vi "nanocal -- nuclear schottky fit -- 2x2 -- V9.vi"() -> ()   [LabVIEW 2021] (continued)
  in  "filenames":u16(ring)=29 caption="files" items=["IDS0183_210310_RAW_cal_CeCoIn5_2nd_071_12T_0.120K_90deg_Tdep_raw_.dat", "IDS0311_210901_RAW_cal_CeCoIn5_4th_040(126)_C(f)_12T_0.120K_45deg_Tdep_raw_.dat", "IDS0359_210907_RAW_cal_CeCoIn5_4th_089_C(f)_12.0T_0.12K_60deg_Tdep_raw_.dat", "IDS0412_220525_RAW_cal_CeCoIn5_5th_017_0T_0deg__fSweep_0.12K_raw_.dat", "IDS0431_220527_RAW_cal_CeCoIn5_5th_036_10T_0deg__fSweep_0.12K_raw_.dat", "IDS0442_220528_RAW_cal_CeCoIn5_5th_047_6T_0deg__fSweep_0.12K_raw_.dat", "IDS0464_220530_RAW_cal_CeCoIn5_5th_069_4T_0deg__fSweep_0.12K_raw_.dat", "IDS0486_220602_RAW_cal_CeCoIn5_5th_091_10T_45deg__fSweep_0.12K_raw_.dat", "IDS0336_210904_RAW_cal_CeCoIn5_4th_065_C(f)_5.0T_0.122K_90deg_Tdep_raw_.dat", "IDS0346_210904_RAW_cal_CeCoIn5_4th_075_C(f)_8.0T_0.122K_90deg_Tdep_raw_.dat", "IDS0378_210909_RAW_cal_CeCoIn5_4th_108_C(f)_8.0T_0.122K_0deg_Tdep_raw_.dat", "IDS0158_210310_RAW_cal_CeCoIn5_2nd_047_12T_fsweep_final_0.14K_0deg_Tdep_raw_.dat", "IDS0300_210427_RAW_cal_CeCoIn5_4th_029(113)_C(f)_12T_0.14K_30deg_NEW_Tdep_raw_.dat", "IDS0184_210310_RAW_cal_CeCoIn5_2nd_072_12T_0.148K_90deg_Tdep_raw_.dat", "IDS0210_210310_RAW_cal_CeCoIn5_2nd_098_fsweep_6T_0.148K_Bdep_raw_.dat", "IDS0379_210909_RAW_cal_CeCoIn5_4th_109_C(f)_8.0T_0.148K_0deg_Tdep_raw_.dat", "IDS0360_210907_RAW_cal_CeCoIn5_4th_090_C(f)_12.0T_0.15K_60deg_Tdep_raw_.dat", "IDS0411_220525_RAW_cal_CeCoIn5_5th_016_0T_0deg__fSweep_0.15K_raw_.dat", "IDS0427_220526_RAW_cal_CeCoIn5_5th_032_10T_0deg__fSweep_0.15K_raw_.dat", "IDS0443_220528_RAW_cal_CeCoIn5_5th_048_6T_0deg__fSweep_0.15K_raw_.dat", "IDS0463_220530_RAW_cal_CeCoIn5_5th_068_4T_0deg__fSweep_0.15K_raw_.dat", "IDS0487_220602_RAW_cal_CeCoIn5_5th_092_10T_45deg__fSweep_0.15K_raw_.dat", "IDS0310_210901_RAW_cal_CeCoIn5_4th_039(125)_C(f)_12T_0.157K_45deg_Tdep_raw_.dat", "IDS0337_210904_RAW_cal_CeCoIn5_4th_066_C(f)_5.0T_0.157K_90deg_Tdep_raw_.dat", "IDS0347_210906_RAW_cal_CeCoIn5_4th_076_C(f)_8.0T_0.157K_90deg_Tdep_raw_.dat", "IDS0305_210831_RAW_cal_CeCoIn5_4th_034(110)_C(f)_12T_0.16K_30deg_NEW_Tdep_raw_.dat", "IDS0361_210908_RAW_cal_CeCoIn5_4th_091_C(f)_12.0T_0.168K_60deg_Tdep_raw_.dat", "IDS0380_210909_RAW_cal_CeCoIn5_4th_110_C(f)_8.0T_0.168K_0deg_Tdep_raw_.dat", "IDS0159_210310_RAW_cal_CeCoIn5_2nd_048_12T_fsweep_0.17K_0deg_Tdep_raw_.dat", "IDS0304_210831_RAW_cal_CeCoIn5_4th_033(112)_C(f)_12T_0.17K_30deg_NEW_Tdep_raw_.dat", "IDS0312_210901_RAW_cal_CeCoIn5_4th_041(127)_C(f)_12T_0.170K_45deg_Tdep_raw_.dat", "IDS0338_210904_RAW_cal_CeCoIn5_4th_067_C(f)_5.0T_0.170K_90deg_Tdep_raw_.dat", "IDS0410_220525_RAW_cal_CeCoIn5_5th_015_0T_0deg__fSweep_0.17K_raw_.dat", "IDS0432_220527_RAW_cal_CeCoIn5_5th_037_10T_0deg__fSweep_0.17K_raw_.dat", "IDS0444_220528_RAW_cal_CeCoIn5_5th_049_6T_0deg__fSweep_0.17K_raw_.dat", "IDS0462_220530_RAW_cal_CeCoIn5_5th_067_4T_0deg__fSweep_0.17K_raw_.dat", "IDS0485_220601_RAW_cal_CeCoIn5_5th_090_10T_45deg__fSweep_0.17K_raw_.dat", "IDS0348_210906_RAW_cal_CeCoIn5_4th_077_C(f)_8.0T_0.178K_90deg_Tdep_raw_.dat", "IDS0181_210310_RAW_cal_CeCoIn5_2nd_070_12T_0.179K_90deg_fsweep_Tdep_raw_.dat", "IDS0424_220526_RAW_cal_CeCoIn5_5th_029_10T_0deg__fSweep_0.19K_raw_.dat", "IDS0185_210310_RAW_cal_CeCoIn5_2nd_073_12T_0.197K_90deg_Tdep_raw_.dat", "IDS0208_210310_RAW_cal_CeCoIn5_2nd_096_Hsweep_0.197K_Bdep_raw_.dat", "IDS0209_210310_RAW_cal_CeCoIn5_2nd_097_Hsweep_0.197K_Bdep_raw_.dat", "IDS0211_210310_RAW_cal_CeCoIn5_2nd_099_fsweep_9T_0.197K_Bdep_raw_.dat", "IDS0212_210310_RAW_cal_CeCoIn5_2nd_100_fsweep_11T_0.197K_Bdep_raw_.dat", "IDS0213_210310_RAW_cal_CeCoIn5_2nd_101_fsweep_10T_0.197K_Bdep_raw_.dat", "IDS0214_210310_RAW_cal_CeCoIn5_2nd_102_fsweep_8T_0.197K_Bdep_raw_.dat", "IDS0215_210310_RAW_cal_CeCoIn5_2nd_103_fsweep_7T_0.197K_Bdep_raw_.dat", "IDS0216_210310_RAW_cal_CeCoIn5_2nd_104_fsweep_5T_0.197K_Bdep_raw_.dat", "IDS0217_210310_RAW_cal_CeCoIn5_2nd_105_fsweep_0T_0.197K_Bdep_raw_.dat", "IDS0330_210901_RAW_cal_CeCoIn5_4th_059_C(f)_1T_0.197K_90deg_Bdep_raw_.dat", "IDS0331_210901_RAW_cal_CeCoIn5_4th_060_C(f)_2T_0.197K_90deg_Bdep_raw_.dat", "IDS0335_210904_RAW_cal_CeCoIn5_4th_064_C(f)_5.0T_0.197K_90deg_Tdep_raw_.dat", "IDS0362_210908_RAW_cal_CeCoIn5_4th_092_C(f)_12.0T_0.197K_60deg_Tdep_raw_.dat", "IDS0377_210909_RAW_cal_CeCoIn5_4th_107_C(f)_8.0T_0.197K_0deg_Tdep_raw_.dat", "IDS0160_210310_RAW_cal_CeCoIn5_2nd_049_12T_fsweep_0.20K_0deg_Tdep_raw_.dat", "IDS0303_210831_RAW_cal_CeCoIn5_4th_032(114)_C(f)_12T_0.20K_30deg_NEW_Tdep_raw_.dat", "IDS0313_210901_RAW_cal_CeCoIn5_4th_042(128)_C(f)_12T_0.200K_45deg_Tdep_raw_.dat", "IDS0349_210906_RAW_cal_CeCoIn5_4th_078_C(f)_8.0T_0.20K_90deg_Tdep_raw_.dat", "IDS0407_220525_RAW_cal_CeCoIn5_5th_012_0T_0deg__fSweep_0.20K_raw_.dat", "IDS0441_220527_RAW_cal_CeCoIn5_5th_045_6T_0deg__fSweep_0.20K_raw_.dat", "IDS0458_220529_RAW_cal_CeCoIn5_5th_063_4T_0deg__fSweep_0.20K_raw_.dat", "IDS0477_220601_RAW_cal_CeCoIn5_5th_082_10T_45deg__fSweep_0.20K_raw_.dat", "IDS0161_210310_RAW_cal_CeCoIn5_2nd_050_12T_fsweep_0.22K_0deg_Tdep_raw_.dat", "IDS0186_210310_RAW_cal_CeCoIn5_2nd_074_12T_0.249K_90deg_Tdep_raw_.dat", "IDS0302_210831_RAW_cal_CeCoIn5_4th_031(115)_C(f)_12T_0.25K_30deg_NEW_Tdep_raw_.dat", "IDS0363_210908_RAW_cal_CeCoIn5_4th_093_C(f)_12.0T_0.25K_60deg_Tdep_raw_.dat", "IDS0381_210909_RAW_cal_CeCoIn5_4th_111_C(f)_8.0T_0.25K_0deg_Tdep_raw_.dat", "IDS0408_220525_RAW_cal_CeCoIn5_5th_013_0T_0deg__fSweep_0.25K_raw_.dat", "IDS0425_220526_RAW_cal_CeCoIn5_5th_030_10T_0deg__fSweep_0.25K_raw_.dat", "IDS0445_220528_RAW_cal_CeCoIn5_5th_050_6T_0deg__fSweep_0.25K_raw_.dat", "IDS0459_220529_RAW_cal_CeCoIn5_5th_064_4T_0deg__fSweep_0.25K_raw_.dat", "IDS0478_220601_RAW_cal_CeCoIn5_5th_083_10T_45deg__fSweep_0.25K_raw_.dat", "IDS0314_210901_RAW_cal_CeCoIn5_4th_043(129)_C(f)_12T_0.255K_45deg_Tdep_raw_.dat", "IDS0339_210904_RAW_cal_CeCoIn5_4th_068_C(f)_5.0T_0.255K_90deg_Tdep_raw_.dat", "IDS0350_210906_RAW_cal_CeCoIn5_4th_079_C(f)_8.0T_0.26K_90deg_Tdep_raw_.dat", "IDS0162_210310_RAW_cal_CeCoIn5_2nd_051_12T_fsweep_0.28K_0deg_Tdep_raw_.dat", "IDS0187_210310_RAW_cal_CeCoIn5_2nd_075_12T_0.300K_90deg_Tdep_raw_.dat", "IDS0301_210831_RAW_cal_CeCoIn5_4th_030(116)_C(f)_12T_0.30K_30deg_NEW_Tdep_raw_.dat", "IDS0315_210901_RAW_cal_CeCoIn5_4th_044(130)_C(f)_12T_0.300K_45deg_Tdep_raw_.dat", "IDS0382_210909_RAW_cal_CeCoIn5_4th_112_C(f)_8.0T_0.30K_0deg_Tdep_raw_.dat", "IDS0409_220525_RAW_cal_CeCoIn5_5th_014_0T_0deg__fSweep_0.30K_raw_.dat", "IDS0426_220526_RAW_cal_CeCoIn5_5th_031_10T_0deg__fSweep_0.30K_raw_.dat", "IDS0446_220528_RAW_cal_CeCoIn5_5th_051_6T_0deg__fSweep_0.30K_raw_.dat", "IDS0460_220529_RAW_cal_CeCoIn5_5th_065_4T_0deg__fSweep_0.30K_raw_.dat", "IDS0479_220601_RAW_cal_CeCoIn5_5th_084_10T_45deg__fSweep_0.30K_raw_.dat", "IDS0364_210908_RAW_cal_CeCoIn5_4th_094_C(f)_12.0T_0.307K_60deg_Tdep_raw_.dat", "IDS0340_210904_RAW_cal_CeCoIn5_4th_069_C(f)_5.0T_0.308K_90deg_Tdep_raw_.dat", "IDS0351_210906_RAW_cal_CeCoIn5_4th_080_C(f)_8.0T_0.31K_90deg_Tdep_raw_.dat", "IDS0163_210310_RAW_cal_CeCoIn5_2nd_052_12T_fsweep_0.33K_0deg_Tdep_raw_.dat", "IDS0188_210310_RAW_cal_CeCoIn5_2nd_076_12T_0.360K_90deg_Tdep_raw_.dat", "IDS0299_210427_RAW_cal_CeCoIn5_4th_028(117)_C(f)_12T_0.36K_30deg_NEW_Tdep_raw_.dat", "IDS0316_210901_RAW_cal_CeCoIn5_4th_045(131)_C(f)_12T_0.360K_45deg_Tdep_raw_.dat", "IDS0341_210904_RAW_cal_CeCoIn5_4th_070_C(f)_5.0T_0.360K_90deg_Tdep_raw_.dat", "IDS0352_210906_RAW_cal_CeCoIn5_4th_081_C(f)_8.0T_0.36K_90deg_Tdep_raw_.dat", "IDS0365_210908_RAW_cal_CeCoIn5_4th_095_C(f)_12.0T_0.36K_60deg_Tdep_raw_.dat", "IDS0383_210910_RAW_cal_CeCoIn5_4th_113_C(f)_8.0T_0.36K_0deg_Tdep_raw_.dat", "IDS0413_220525_RAW_cal_CeCoIn5_5th_018_0T_0deg__fSweep_0.36K_raw_.dat", "IDS0428_220526_RAW_cal_CeCoIn5_5th_033_10T_0deg__fSweep_0.36K_raw_.dat", "IDS0447_220528_RAW_cal_CeCoIn5_5th_052_6T_0deg__fSweep_0.36K_raw_.dat", "IDS0461_220529_RAW_cal_CeCoIn5_5th_066_4T_0deg__fSweep_0.36K_raw_.dat", "IDS0480_220601_RAW_cal_CeCoIn5_5th_085_10T_45deg__fSweep_0.36K_raw_.dat", "IDS0164_210310_RAW_cal_CeCoIn5_2nd_053_12T_fsweep_0.40K_0deg_Tdep_raw_.dat", "IDS0429_220526_RAW_cal_CeCoIn5_5th_034_10T_0deg__fSweep_0.42K_raw_.dat", "IDS0448_220528_RAW_cal_CeCoIn5_5th_053_6T_0deg__fSweep_0.42K_raw_.dat", "IDS0481_220601_RAW_cal_CeCoIn5_5th_086_10T_45deg__fSweep_0.42K_raw_.dat", "IDS0189_210310_RAW_cal_CeCoIn5_2nd_077_12T_0.430K_90deg_Tdep_raw_.dat", "IDS0298_210427_RAW_cal_CeCoIn5_4th_027(118)_C(f)_12T_0.43K_30deg_NEW_Tdep_raw_.dat", "IDS0317_210901_RAW_cal_CeCoIn5_4th_046(132)_C(f)_12T_0.43K_45deg_Tdep_raw_.dat", "IDS0366_210908_RAW_cal_CeCoIn5_4th_096_C(f)_12.0T_0.43K_60deg_Tdep_raw_.dat", "IDS0384_210910_RAW_cal_CeCoIn5_4th_114_C(f)_8.0T_0.43K_0deg_Tdep_raw_.dat", "IDS0414_220525_RAW_cal_CeCoIn5_5th_019_0T_0deg__fSweep_0.43K_raw_.dat", "IDS0465_220530_RAW_cal_CeCoIn5_5th_070_4T_0deg__fSweep_0.43K_raw_.dat", "IDS0342_210904_RAW_cal_CeCoIn5_4th_071_C(f)_5.0T_0.438K_90deg_Tdep_raw_.dat", "IDS0353_210906_RAW_cal_CeCoIn5_4th_082_C(f)_8.0T_0.438K_90deg_Tdep_raw_.dat", "IDS0165_210310_RAW_cal_CeCoIn5_2nd_054_12T_fsweep_0.48K_0deg_Tdep_raw_.dat", "IDS0190_210310_RAW_cal_CeCoIn5_2nd_078_12T_0.512K_90deg_Tdep_raw_.dat", "IDS0430_220526_RAW_cal_CeCoIn5_5th_035_10T_0deg__fSweep_0.52K_raw_.dat", "IDS0449_220528_RAW_cal_CeCoIn5_5th_054_6T_0deg__fSweep_0.52K_raw_.dat", "IDS0482_220601_RAW_cal_CeCoIn5_5th_087_10T_45deg__fSweep_0.52K_raw_.dat", "IDS0297_210427_RAW_cal_CeCoIn5_4th_026(119)_C(f)_12T_0.53K_30deg_NEW_Tdep_raw_.dat", "IDS0318_210901_RAW_cal_CeCoIn5_4th_047(133)_C(f)_12T_0.53K_45deg_Tdep_raw_.dat", "IDS0343_210904_RAW_cal_CeCoIn5_4th_072_C(f)_5.0T_0.53K_90deg_Tdep_raw_.dat", "IDS0354_210906_RAW_cal_CeCoIn5_4th_083_C(f)_8.0T_0.53K_90deg_Tdep_raw_.dat", "IDS0367_210908_RAW_cal_CeCoIn5_4th_097_C(f)_12.0T_0.53K_60deg_Tdep_raw_.dat", "IDS0385_210910_RAW_cal_CeCoIn5_4th_115_C(f)_8.0T_0.53K_0deg_Tdep_raw_.dat", "IDS0415_220525_RAW_cal_CeCoIn5_5th_020_0T_0deg__fSweep_0.53K_raw_.dat", "IDS0466_220530_RAW_cal_CeCoIn5_5th_071_4T_0deg__fSweep_0.53K_raw_.dat", "IDS0166_210310_RAW_cal_CeCoIn5_2nd_055_12T_fsweep_0.58K_0deg_Tdep_raw_.dat", "IDS0191_210310_RAW_cal_CeCoIn5_2nd_079_12T_0.610K_90deg_Tdep_raw_.dat", "IDS0296_210427_RAW_cal_CeCoIn5_4th_025(120)_C(f)_12T_0.62K_30deg_NEW_Tdep_raw_.dat", "IDS0319_210901_RAW_cal_CeCoIn5_4th_048(134)_C(f)_12T_0.62K_45deg_Tdep_raw_.dat", "IDS0344_210904_RAW_cal_CeCoIn5_4th_073_C(f)_5.0T_0.62K_90deg_Tdep_raw_.dat", "IDS0433_220527_RAW_cal_CeCoIn5_5th_038_10T_0deg__fSweep_0.62K_raw_.dat", "IDS0450_220528_RAW_cal_CeCoIn5_5th_055_6T_0deg__fSweep_0.62K_raw_.dat", "IDS0467_220530_RAW_cal_CeCoIn5_5th_072_4T_0deg__fSweep_0.62K_raw_.dat", "IDS0483_220601_RAW_cal_CeCoIn5_5th_088_10T_45deg__fSweep_0.62K_raw_.dat", "IDS0368_210908_RAW_cal_CeCoIn5_4th_098_C(f)_12.0T_0.63K_60deg_Tdep_raw_.dat", "IDS0386_210910_RAW_cal_CeCoIn5_4th_116_C(f)_8.0T_0.63K_0deg_Tdep_raw_.dat", "IDS0416_220525_RAW_cal_CeCoIn5_5th_021_0T_0deg__fSweep_0.63K_raw_.dat", "IDS0220_210310_RAW_cal_CeCoIn5_2nd_108_fsweep_0T_0.677K_Bdep_raw_.dat", "IDS0167_210310_RAW_cal_CeCoIn5_2nd_056_12T_fsweep_0.68K_0deg_Tdep_raw_.dat", "IDS0192_210310_RAW_cal_CeCoIn5_2nd_080_12T_0.810K_90deg_Tdep_raw_.dat", "IDS0434_220527_RAW_cal_CeCoIn5_5th_039_10T_0deg__fSweep_0.82K_raw_.dat", "IDS0451_220528_RAW_cal_CeCoIn5_5th_056_6T_0deg__fSweep_0.82K_raw_.dat", "IDS0468_220530_RAW_cal_CeCoIn5_5th_073_4T_0deg__fSweep_0.82K_raw_.dat", "IDS0484_220601_RAW_cal_CeCoIn5_5th_089_10T_45deg__fSweep_0.82K_raw_.dat", "IDS0295_210427_RAW_cal_CeCoIn5_4th_024(121)_C(f)_12T_0.83K_30deg_NEW_Tdep_raw_.dat", "IDS0320_210901_RAW_cal_CeCoIn5_4th_049(135)_C(f)_12T_0.83K_45deg_Tdep_raw_.dat", "IDS0355_210906_RAW_cal_CeCoIn5_4th_085_C(f)_8.0T_0.83K_90deg_Tdep_raw_.dat", "IDS0369_210908_RAW_cal_CeCoIn5_4th_099_C(f)_12.0T_0.83K_60deg_Tdep_raw_.dat", "IDS0387_210910_RAW_cal_CeCoIn5_4th_117_C(f)_8.0T_0.83K_0deg_Tdep_raw_.dat", "IDS0417_220525_RAW_cal_CeCoIn5_5th_022_0T_0deg__fSweep_0.83K_raw_.dat", "IDS0168_210310_RAW_cal_CeCoIn5_2nd_057_12T_fsweep_0.91K_0deg_Tdep_raw_.dat", "IDS0219_210310_RAW_cal_CeCoIn5_2nd_107_fsweep_0T_1.0K_Bdep_raw_.dat", "IDS0193_210310_RAW_cal_CeCoIn5_2nd_081_12T_1.1K_90deg_Tdep_raw_.dat", "IDS0418_220525_RAW_cal_CeCoIn5_5th_023_0T_0deg__fSweep_1.12K_raw_.dat", "IDS0435_220527_RAW_cal_CeCoIn5_5th_040_10T_0deg__fSweep_1.12K_raw_.dat", "IDS0452_220528_RAW_cal_CeCoIn5_5th_057_6T_0deg__fSweep_1.12K_raw_.dat", "IDS0469_220530_RAW_cal_CeCoIn5_5th_074_4T_0deg__fSweep_1.12K_raw_.dat", "IDS0488_220602_RAW_cal_CeCoIn5_5th_093_10T_45deg__fSweep_1.12K_raw_.dat", "IDS0294_210427_RAW_cal_CeCoIn5_4th_023(122)_C(f)_12T_1.13K_30deg_NEW_Tdep_raw_.dat", "IDS0321_210901_RAW_cal_CeCoIn5_4th_050(136)_C(f)_12T_1.13K_45deg_Tdep_raw_.dat", "IDS0370_210908_RAW_cal_CeCoIn5_4th_100_C(f)_12.0T_1.13K_60deg_Tdep_raw_.dat", "IDS0388_210910_RAW_cal_CeCoIn5_4th_118_C(f)_8.0T_1.13K_0deg_Tdep_raw_.dat", "IDS0169_210310_RAW_cal_CeCoIn5_2nd_058_12T_fsweep_1.23K_0deg_Tdep_raw_.dat", "IDS0391_210910_RAW_cal_CeCoIn5_4th_121_C(f)_8.0T_1.25K_0deg_Tdep_raw_.dat", "IDS0439_220527_RAW_cal_CeCoIn5_5th_044_10T_0deg__fSweep_1.28K_raw_.dat", "IDS0395_210910_RAW_cal_CeCoIn5_4th_125_C(f)_8.0T_1.31K_0deg_Tdep_raw_.dat", "IDS0392_210910_RAW_cal_CeCoIn5_4th_122_C(f)_8.0T_1.39K_0deg_Tdep_raw_.dat", "IDS0389_210910_RAW_cal_CeCoIn5_4th_119_C(f)_8.0T_1.52K_0deg_Tdep_raw_.dat", "IDS0218_210310_RAW_cal_CeCoIn5_2nd_106_fsweep_0T_1.55K_Bdep_raw_.dat", "IDS0453_220529_RAW_cal_CeCoIn5_5th_058_6T_0deg__fSweep_1.70K_raw_.dat", "IDS0194_210310_RAW_cal_CeCoIn5_2nd_082_12T_1.8K_90deg_Tdep_raw_.dat", "IDS0293_210427_RAW_cal_CeCoIn5_4th_022(123)_C(f)_12T_1.90K_30deg_NEW_Tdep_raw_.dat", "IDS0322_210901_RAW_cal_CeCoIn5_4th_051(137)_C(f)_12T_1.90K_45deg_Tdep_raw_.dat", "IDS0371_210908_RAW_cal_CeCoIn5_4th_101_C(f)_12.0T_1.90K_60deg_Tdep_raw_.dat", "IDS0390_210910_RAW_cal_CeCoIn5_4th_120_C(f)_8.0T_1.90K_0deg_Tdep_raw_.dat", "IDS0419_220525_RAW_cal_CeCoIn5_5th_024_0T_0deg__fSweep_1.90K_raw_.dat", "IDS0436_220527_RAW_cal_CeCoIn5_5th_041_10T_0deg__fSweep_1.90K_raw_.dat", "IDS0454_220529_RAW_cal_CeCoIn5_5th_059_6T_0deg__fSweep_1.90K_raw_.dat", "IDS0470_220530_RAW_cal_CeCoIn5_5th_075_4T_0deg__fSweep_1.90K_raw_.dat", "IDS0489_220602_RAW_cal_CeCoIn5_5th_094_10T_45deg__fSweep_1.90K_raw_.dat", "IDS0170_210310_RAW_cal_CeCoIn5_2nd_059_12T_fsweep_1.97K_0deg_Tdep_raw_.dat", "IDS0420_220525_RAW_cal_CeCoIn5_5th_025_0T_0deg__fSweep_2.10K_raw_.dat", "IDS0421_220525_RAW_cal_CeCoIn5_5th_026_0T_0deg__fSweep_2.30K_raw_.dat", "IDS0471_220530_RAW_cal_CeCoIn5_5th_076_4T_0deg__fSweep_2.30K_raw_.dat", "IDS0195_210310_RAW_cal_CeCoIn5_2nd_083_12T_3.0K_90deg_Tdep_raw_.dat", "IDS0472_220530_RAW_cal_CeCoIn5_5th_077_4T_0deg__fSweep_3.07K_raw_.dat", "IDS0306_210831_RAW_cal_CeCoIn5_4th_035(124)_C(f)_12T_3.10K_30deg_NEW_Tdep_raw_.dat", "IDS0323_210901_RAW_cal_CeCoIn5_4th_052(138)_C(f)_12T_3.10K_45deg_Tdep_raw_.dat", "IDS0422_220525_RAW_cal_CeCoIn5_5th_027_0T_0deg__fSweep_3.10K_raw_.dat", "IDS0437_220527_RAW_cal_CeCoIn5_5th_042_10T_0deg__fSweep_3.10K_raw_.dat", "IDS0455_220529_RAW_cal_CeCoIn5_5th_060_6T_0deg__fSweep_3.10K_raw_.dat", "IDS0490_220602_RAW_cal_CeCoIn5_5th_095_10T_45deg__fSweep_3.10K_raw_.dat", "IDS0372_210908_RAW_cal_CeCoIn5_4th_102_C(f)_12.0T_3.11K_60deg_Tdep_raw_.dat", "IDS0393_210910_RAW_cal_CeCoIn5_4th_123_C(f)_8.0T_3.11K_0deg_Tdep_raw_.dat", "IDS0171_210310_RAW_cal_CeCoIn5_2nd_060_12T_fsweep_3.19K_0deg_Tdep_raw_.dat", "IDS0196_210310_RAW_cal_CeCoIn5_2nd_084_12T_5.7K_90deg_Tdep_raw_.dat", "IDS0324_210901_RAW_cal_CeCoIn5_4th_053(139)_C(f)_12T_5.70K_45deg_Tdep_raw_.dat", "IDS0438_220527_RAW_cal_CeCoIn5_5th_043_10T_0deg__fSweep_5.70K_raw_.dat", "IDS0456_220529_RAW_cal_CeCoIn5_5th_061_6T_0deg__fSweep_5.70K_raw_.dat", "IDS0473_220531_RAW_cal_CeCoIn5_5th_078_4T_0deg__fSweep_5.70K_raw_.dat", "IDS0373_210908_RAW_cal_CeCoIn5_4th_103_C(f)_12.0T_5.75K_60deg_Tdep_raw_.dat", "IDS0394_210910_RAW_cal_CeCoIn5_4th_124_C(f)_8.0T_5.75K_0deg_Tdep_raw_.dat", "IDS0172_210310_RAW_cal_CeCoIn5_2nd_061_12T_fsweep_5.8K_0deg_Tdep_raw_.dat"]
  in  "folder":path=path "/opt/new/Dropbox/shared_AkashAndreas/paper-CeCoIn5/Original RAW data"
  in  "file pattern":string="IDS*RAW*_raw_.dat"
  in  "string IN → Math!":bool
  in  "Math→ string OUT! :s":bool
  out "string OUT":string="  \"IDS0158_210310_RAW_cal__ref_\" ->   <|    \"ζ\" -> 0.338724462580   ,  \"τ1\" -> 0.031757745266   ,  \"τS\" -> 0.247286819047   ,  \"τN\" -> 0.322740818116   ,  \"τC\" -> 0.001034291318   ,  \"κ0\" -> 0.000000000505   ,  \"mm1\" -> 0.000261080239   ,  \"mm2\" -> 0.013473055910   ,  \"mm3\" -> 0.782167842652   ,  \"T\" -> 0.140000000000   ,  \"B\" -> 12.000000000000   ,  \"θ\" -> 0.000000000000   ,  \"Reoff\" -> -114641566.265060246000   ,  \"Imoff\" -> 0.000000000000   ,  \"στ1\" -> 0.023975320210   ,  \"στS\" -> 0.076414054009   ,  \"στN\" -> 0.076454917520    |>   , \r\"IDS0158_210310_RAW_cal__sam_\" ->   <|    \"ζ\" -> 0.286336668596   ,  \"τ1\" -> 0.037477267671   ,  \"τS\" -> 0.354459287884   ,  \"τN\" -> 0.444916383639   ,  \"τC\" -> 0.001225600579   ,  \"κ0\" -> 0.000000000596   ,  \"mm1\" -> 0.000272242393   ,  \"mm2\" -> 0.016302418461   ,  \"mm3\" -> 1.050394445660   ,  \"T\" -> 0.140000000000   ,  \"B\" -> 12.000000000000   ,  \"θ\" -> 0.000000000000   ,  \"Reoff\" -> 0.000000000000   ,  \"Imoff\" -> 0.000000000000   ,  \"στ1\" -> 0.000000000000   ,  \"στS\" -> 0.000000000000   ,  \"στN\" -> 0.000000000000    |>   , \r\"IDS0159_210310_RAW_cal__ref_\" ->   <|    \"ζ\" -> 0.271267920492   ,  \"τ1\" -> 0.029985631647   ,  \"τS\" -> 0.193691005295   ,  \"τN\" -> 0.182171075098   ,  \"τC\" -> 0.001008816819   ,  \"κ0\" -> 0.000000000648   ,  \"mm1\" -> 0.000214568285   ,  \"mm2\" -> 0.015007137955   ,  \"mm3\" -> 0.493594147559   ,  \"T\" -> 0.170000000000   ,  \"B\" -> 12.000000000000   ,  \"θ\" -> 0.000000000000   ,  \"Reoff\" -> -68518072.289156615700   ,  \"Imoff\" -> 0.000000000000   ,  \"στ1\" -> 0.012908928279   ,  \"στS\" -> 0.012278249433   ,  \"στN\" -> 0.000000000000    |>   , \r\"IDS0159_210310_RAW_cal__sam_\" ->   <|    \"ζ\" -> 0.219100303741   ,  \"τ1\" -> 0.028643012604   ,  \"τS\" -> 0.279362928811   ,  \"τN\" -> 0.246156444058   ,  \"τC\" -> 0.001272401549   ,  \"κ0\" -> 0.000000000760   ,  \"mm1\" -> 0.000227975653   ,  \"mm2\" -> 0.014929571562   ,  \"mm3\" -> 0.655418694024   ,  \"T\" -> 0.170000000000   ,  \"B\" -> 12.000000000000   ,  \"θ\" -> 0.000000000000   ,  \"Reoff\" -> 0.000000000000   ,  \"Imoff\" -> 0.000000000000   ,  \"στ1\" -> 0.000000000000   ,  \"στS\" -> 0.000000000000   ,  \"στN\" -> 0.000000000000    |>   , \r\"IDS0160_210310_RAW_cal__ref_\" ->   <|    \"ζ\" -> 0.207139977904   ,  \"τ1\" -> 0.027467343957   ,  \"τS\" -> 0.117438673826   ,  \"τN\" -> 0.102057074143   ,  \"τC\" -> 0.000949663971   ,  \"κ0\" -> 0.000000000917   ,  \"mm1\" -> 0.000162053218   ,  \"mm2\" -> 0.014024936030   ,  \"mm3\" -> 0.279192111033   ,  \"T\" -> 0.200000000000   ,  \"B\" -> 12.000000000000   ,  \"θ\" -> 0.000000000000   ,  \"Reoff\" -> -40668674.698795177000   ,  \"Imoff\" -> 0.000000000000   ,  \"στ1\" -> 0.009618369087   ,  \"στS\" -> 0.007137384425   ,  \"στN\" -> 0.000000000000    |>   , \r\"IDS0160_210310_RAW_cal__sam_\" ->   <|    \"ζ\" -> 0.170488637524   ,  \"τ1\" -> 0.029234231120   ,  \"τS\" -> 0.149095458227   ,  \"τN\" -> 0.151792620275   ,  \"τC\" -> 0.001113424175   ,  \"κ0\" -> 0.000000001042   ,  \"mm1\" -> 0.000161291869   ,  \"mm2\" -> 0.013922632736   ,  \"mm3\" -> 0.368449807743   ,  \"T\" -> 0.200000000000   ,  \"B\" -> 12.000000000000   ,  \"θ\" -> 0.000000000000   ,  \"Reoff\" -> 0.000000000000   ,  \"Imoff\" -> 0.000000000000   ,  \"στ1\" -> 0.000000000000   ,  \"στS\" -> 0.000000000000   ,  \"στN\" -> 0.000000000000    |>   , \r\"IDS0161_210310_RAW_cal__ref_\" ->   <|    \"ζ\" -> 0.165651103495   ,  \"τ1\" -> 0.025219369633   ,  \"τS\" -> 0.095243887499   ,  \"τN\" -> 0.068405844588   ,  \"τC\" -> 0.001096621932   ,  \"κ0\" -> 0.000000001058   ,  \"mm1\" -> 0.000154524257   ,  \"mm2\" -> 0.013909362731   ,  \"mm3\" -> 0.203010595371   ,  \"T\" -> 0.220000000000   ,  \"B\" -> 12.000000000000   ,  \"θ\" -> 0.000000000000   ,  \"Reoff\" -> -26138554.216867461800   ,  \"Imoff\" -> 0.000000000000   ,  \"στ1\" -> 0.007587881902   ,  \"στS\" -> 0.004844828321   ,  \"στN\" -> 0.000000000000    |>   , \r\"IDS0161_210310_RAW_cal__sam_\" ->   <|    \"ζ\" -> 0.130531197151   ,  \"τ1\" -> 0.025704482770   ,  \"τS\" -> 0.129606657196   ,  \"τN\" -> 0.091602369165   ,  \"τC\" -> 0.001441379995   ,  \"κ0\" -> 0.000000001211   ,  \"mm1\" -> 0.000164978070   ,  \"mm2\" -> 0.014468182937   ,  \"mm3\" -> 0.262596407151   ,  \"T\" -> 0.220000000000   ,  \"B\" -> 12.000000000000   ,  \"θ\" -> 0.000000000000   ,  \"Reoff\" -> 0.000000000000   ,  \"Imoff\" -> 0.000000000000   ,  \"στ1\" -> 0.000000000000   ,  \"στS\" -> 0.000000000000   ,  \"στN\" -> 0.000000000000    |>   , \r\"IDS0162_210310_RAW_cal__ref_\" ->   <|    \"ζ\" -> 0.096222034275   ,  \"τ1\" -> 0.023686784650   ,  \"τS\" -> 0.070336744639   ,  \"τN\" -> 0.023939989572   ,  \"τC\" -> 0.001388596335   ,  \"κ0\" -> 0.000000001367   ,  \"mm1\" -> 0.000119909077   ,  \"mm2\" -> 0.016622969082   ,  \"mm3\" -> 0.111680736187   ,  \"T\" -> 0.280000000000   ,  \"B\" -> 12.000000000000   ,  \"θ\" -> 0.000000000000   ,  \"Reoff\" -> -11003012.048192769300   ,  \"Imoff\" -> 0.000000000000   ,  \"στ1\" -> 0.008753356754   ,  \"στS\" -> 0.002669913437   ,  \"στN\" -> 0.000000000000    |>   , \r\"IDS0162_210310_RAW_cal__sam_\" ->   <|    \"ζ\" -> 0.078258046754   ,  \"τ1\" -> 0.028009840731   ,  \"τS\" -> 0.092122038762   ,  \"τN\" -> 0.030129595899   ,  \"τC\" -> 0.001641062244   ,  \"κ0\" -> 0.000000001543   ,  \"mm1\" -> 0.000117303440   ,  \"mm2\" -> 0.019983073008   ,  \"mm3\" -> 0.141369335330   ,  \"T\" -> 0.280000000000   ,  \"B\" -> 12.000000000000   ,  \"θ\" -> 0.000000000000   ,  \"Reoff\" -> 0.000000000000   ,  \"Imoff\" -> 0.000000000000   ,  \"στ1\" -> 0.000000000000   ,  \"στS\" -> 0.000000000000   ,  \"στN\" -> 0.000000000000    |>   , \r\"IDS0163_210310_RAW_cal__ref_\" ->   <|    \"ζ\" -> 0.066672200447   ,  \"τ1\" -> 0.021639337174   ,  \"τS\" -> 0.054330230678   ,  \"τN\" -> 0.012190158529   ,  \"τC\" -> 0.001673698086   ,  \"κ0\" -> 0.000000001744   ,  \"mm1\" -> 0.000101848885   ,  \"mm2\" -> 0.016608176692   ,  \"mm3\" -> 0.077558459612   ,  \"T\" -> 0.330000000000   ,  \"B\" -> 12.000000000000   ,  \"θ\" -> 0.000000000000   ,  \"Reoff\" -> -6192771.084337353710   ,  \"Imoff\" -> 0.000000000000   ,  \"στ1\" -> 0.010795838687   ,  \"στS\" -> 0.002003612837   ,  \"στN\" -> 0.000000000000    |>   , \r\"IDS0163_210310_RAW_cal__sam_\" ->   <|    \"ζ\" -> 0.054088186012   ,  \"τ1\" -> 0.023838802615   ,  \"τS\" -> 0.069079396629   ,  \"τN\" -> 0.016435267456   ,  \"τC\" -> 0.002025071743   ,  \"κ0\" -> 0.000000001955   ,  \"mm1\" -> 0.000101234646   ,  \"mm2\" -> 0.018244822177   ,  \"mm3\" -> 0.097657814678   ,  \"T\" -> 0.330000000000   ,  \"B\" -> 12.000000000000   ,  \"θ\" -> 0.000000000000   ,  \"Reoff\" -> 0.000000000000   ,  \"Imoff\" -> 0.000000000000   ,  \"στ1\" -> 0.000000000000   ,  \"στS\" -> 0.000000000000   ,  \"στN\" -> 0.000000000000    |>   , \r\"IDS0164_210310_RAW_cal__ref_\" ->   <|    \"ζ\" -> 0.047185670549   ,  \"τ1\" -> 0.020999787986   ,  \"τS\" -> 0.044123234525   ,  \"τN\" -> 0.006414229914   ,  \"τC\" -> 0.002330922094   ,  \"κ0\" -> 0.000000002161   ,  \"mm1\" -> 0.000100189786   ,  \"mm2\" -> 0.017276594586   ,  \"mm3\" -> 0.058876034294   ,  \"T\" -> 0.400000000000   ,  \"B\" -> 12.000000000000   ,  \"θ\" -> 0.000000000000   ,  \"Reoff\" -> -3126506.024096369740   ,  \"Imoff\" -> 0.000000000000   ,  \"στ1\" -> 0.014319461595   ,  \"στS\" -> 0.001588428387   ,  \"στN\" -> 0.000000000000    |>   , \r\"IDS0164_210310_RAW_cal__sam_\" ->   <|    \"ζ\" -> 0.039314966212   ,  \"τ1\" -> 0.020712803909   ,  \"τS\" -> 0.055413767550   ,  \"τN\" -> 0.008474403424   ,  \"τC\" -> 0.002674063387   ,  \"κ0\" -> 0.000000002415   ,  \"mm1\" -> 0.000096818147   ,  \"mm2\" -> 0.017190811405   ,  \"mm3\" -> 0.072499170001   ,  \"T\" -> 0.400000000000   ,  \"B\" -> 12.000000000000   ,  \"θ\" -> 0.000000000000   ,  \"Reoff\" -> 0.000000000000   ,  \"Imoff\" -> 0.000000000000   ,  \"στ1\" -> 0.000000000000   ,  \"στS\" -> 0.000000000000   ,  \"στN\" -> 0.000000000000    |>   , \r\"IDS0165_210310_RAW_cal__ref_\" ->   <|    \"ζ\" -> 0.033577393126   ,  \"τ1\" -> 0.018946820322   ,  \"τS\" -> 0.035749921348   ,  \"τN\" -> 0.004008447047   ,  \"τC\" -> 0.003122429757   ,  \"κ0\" -> 0.000000002680   ,  \"mm1\" -> 0.000093748549   ,  \"mm2\" -> 0.016142439680   ,  \"mm3\" -> 0.046926412611   ,  \"T\" -> 0.480000000000   ,  \"B\" -> 12.000000000000   ,  \"θ\" -> 0.000000000000   ,  \"Reoff\" -> -1313253.012048184870   ,  \"Imoff\" -> 0.000000000000   ,  \"στ1\" -> 0.017565086331   ,  \"στS\" -> 0.001375721175   ,  \"στN\" -> 0.000000000000    |>   , \r\"IDS0165_210310_RAW_cal__sam_\" ->   <|    \"ζ\" -> 0.031945976845   ,  \"τ1\" -> 0.019000922826   ,  \"τS\" -> 0.045624146388   ,  \"τN\" -> 0.005314716063   ,  \"τC\" -> 0.002488383471   ,  \"κ0\" -> 0.000000002954   ,  \"mm1\" -> 0.000073272643   ,  \"mm2\" -> 0.016306894362   ,  \"mm3\" -> 0.057675293464   ,  \"T\" -> 0.480000000000   ,  \"B\" -> 12.000000000000   ,  \"θ\" -> 0.000000000000   ,  \"Reoff\" -> 0.000000000000   ,  \"Imoff\" -> 0.000000000000   ,  \"στ1\" -> 0.000000000000   ,  \"στS\" -> 0.000000000000   ,  \"στN\" -> 0.000000000000    |>   , \r\"IDS0166_210310_RAW_cal__ref_\" ->   <|    \"ζ\" -> 0.026134408941   ,  \"τ1\" -> 0.018837221506   ,  \"τS\" -> 0.029046436266   ,  \"τN\" -> 0.002475934064   ,  \"τC\" -> 0.003637611641   ,  \"κ0\" -> 0.000000003369   ,  \"mm1\" -> 0.000082770074   ,  \"mm2\" -> 0.016386102123   ,  \"mm3\" -> 0.038352149797   ,  \"T\" -> 0.580000000000   ,  \"B\" -> 12.000000000000   ,  \"θ\" -> 0.000000000000   ,  \"Reoff\" -> -406626.506024092435   ,  \"Imoff\" -> 0.000000000000   ,  \"στ1\" -> 0.034768871814   ,  \"στS\" -> 0.001627850434   ,  \"στN\" -> 0.000000000000    |>   , \r\"IDS0166_210310_RAW_cal__sam_\" ->   <|    \"ζ\" -> 0.023031239946   ,  \"τ1\" -> 0.018268814012   ,  \"τS\" -> 0.037269400776   ,  \"τN\" -> 0.002696792890   ,  \"τC\" -> 0.003257395394   ,  \"κ0\" -> 0.000000003720   ,  \"mm1\" -> 0.000067670174   ,  \"mm2\" -> 0.016445281937   ,  \"mm3\" -> 0.045899921957   ,  \"T\" -> 0.580000000000   ,  \"B\" -> 12.000000000000   ,  \"θ\" -> 0.000000000000   ,  \"Reoff\" -> 0.000000000000   ,  \"Imoff\" -> 0.000000000000   ,  \"στ1\" -> 0.000000000000   ,  \"στS\" -> 0.000000000000   ,  \"στN\" -> 0.000000000000    |>   , \r\"IDS0167_210310_RAW_cal__ref_\" ->   <|    \"ζ\" -> 0.026557278794   ,  \"τ1\" -> 0.016933945977   ,  \"τS\" -> 0.022881111855   ,  \"τN\" -> 0.001392473895   ,  \"τC\" -> 0.004119437148   ,  \"κ0\" -> 0.000000003981   ,  \"mm1\" -> 0.000090964667   ,  \"mm2\" -> 0.015177563241   ,  \"mm3\" -> 0.030703081351   ,  \"T\" -> 0.680000000000   ,  \"B\" -> 12.000000000000   ,  \"θ\" -> 0.000000000000   ,  \"Reoff\" -> 0.000000000000   ,  \"Imoff\" -> 0.000000000000   ,  \"στ1\" -> 0.000000000000   ,  \"στS\" -> 0.000000000000   ,  \"στN\" -> 0.000000000000    |>   , \r\"IDS0167_210310_RAW_cal__sam_\" ->   <|    \"ζ\" -> 0.019920170845   ,  \"τ1\" -> 0.016368892412   ,  \"τS\" -> 0.030579536580   ,  \"τN\" -> 0.001736017565   ,  \"τC\" -> 0.004971418152   ,  \"κ0\" -> 0.000000004410   ,  \"mm1\" -> 0.000083939556   ,  \"mm2\" -> 0.015095997595   ,  \"mm3\" -> 0.039119658918   ,  \"T\" -> 0.680000000000   ,  \"B\" -> 12.000000000000   ,  \"θ\" -> 0.000000000000   ,  \"Reoff\" -> 0.000000000000   ,  \"Imoff\" -> 0.000000000000   ,  \"στ1\" -> 0.000000000000   ,  \"στS\" -> 0.000000000000   ,  \"στN\" -> 0.000000000000    |>   , \r\"IDS0168_210310_RAW_cal__ref_\" ->   <|    \"ζ\" -> 0.022041296958   ,  \"τ1\" -> 0.014045615335   ,  \"τS\" -> 0.018889590451   ,  \"τN\" -> 0.000813465770   ,  \"τC\" -> 0.004122617309   ,  \"κ0\" -> 0.000000005540   ,  \"mm1\" -> 0.000073491061   ,  \"mm2\" -> 0.013002629707   ,  \"mm3\" -> 0.025229449010   ,  \"T\" -> 0.910000000000   ,  \"B\" -> 12.000000000000   ,  \"θ\" -> 0.000000000000   ,  \"Reoff\" -> 0.000000000000   ,  \"Imoff\" -> 0.000000000000   ,  \"στ1\" -> 0.000000000000   ,  \"στS\" -> 0.000000000000   ,  \"στN\" -> 0.000000000000    |>   , \r\"IDS0168_210310_RAW_cal__sam_\" ->   <|    \"ζ\" -> 0.017558473054   ,  \"τ1\" -> 0.014545104284   ,  \"τS\" -> 0.022979681288   ,  \"τN\" -> 0.000840829385   ,  \"τC\" -> 0.005228030240   ,  \"κ0\" -> 0.000000006068   ,  \"mm1\" -> 0.000073916527   ,  \"mm2\" -> 0.013750428362   ,  \"mm3\" -> 0.030187552103   ,  \"T\" -> 0.910000000000   ,  \"B\" -> 12.000000000000   ,  \"θ\" -> 0.000000000000   ,  \"Reoff\" -> 0.000000000000   ,  \"Imoff\" -> 0.000000000000   ,  \"στ1\" -> 0.000000000000   ,  \"στS\" -> 0.000000000000   ,  \"στN\" -> 0.000000000000    |>   , \r\"IDS0169_210310_RAW_cal__ref_\" ->   <|    \"ζ\" -> 0.021090283514   ,  \"τ1\" -> 0.013945744068   ,  \"τS\" -> 0.014386606899   ,  \"τN\" -> 0.000345175874   ,  \"τC\" -> 0.004902956629   ,  \"κ0\" -> 0.000000007742   ,  \"mm1\" -> 0.000076221408   ,  \"mm2\" -> 0.013209066715   ,  \"mm3\" -> 0.020605892822   ,  \"T\" -> 1.230000000000   ,  \"B\" -> 12.000000000000   ,  \"θ\" -> 0.000000000000   ,  \"Reoff\" -> 0.000000000000   ,  \"Imoff\" -> 0.000000000000   ,  \"στ1\" -> 0.000000000000   ,  \"στS\" -> 0.000000000000   ,  \"στN\" -> 0.000000000000    |>   , \r\"IDS0169_210310_RAW_cal__sam_\" ->   <|    \"ζ\" -> 0.011916480594   ,  \"τ1\" -> 0.012551282481   ,  \"τS\" -> 0.018233218660   ,  \"τN\" -> 0.000345702746   ,  \"τC\" -> 0.004699451527   ,  \"κ0\" -> 0.000000008451   ,  \"mm1\" -> 0.000044190864   ,  \"mm2\" -> 0.012162820727   ,  \"mm3\" -> 0.023844039179   ,  \"T\" -> 1.230000000000   ,  \"B\" -> 12.000000000000   ,  \"θ\" -> 0.000000000000   ,  \"Reoff\" -> 0.000000000000   ,  \"Imoff\" -> 0.000000000000   ,  \"στ1\" -> 0.000000000000   ,  \"στS\" -> 0.000000000000   ,  \"στN\" -> 0.000000000000    |>   , \r\"IDS0170_210310_RAW_cal__ref_\" ->   <|    \"ζ\" -> 0.021449250230   ,  \"τ1\" -> 0.014564522147   ,  \"τS\" -> 0.008878867204   ,  \"τN\" -> 0.000064984242   ,  \"τC\" -> 0.006207353748   ,  \"κ0\" -> 0.000000012530   ,  \"mm1\" -> 0.000077778127   ,  \"mm2\" -> 0.013872772336   ,  \"mm3\" -> 0.015957015786   ,  \"T\" -> 1.970000000000   ,  \"B\" -> 12.000000000000   ,  \"θ\" -> 0.000000000000   ,  \"Reoff\" -> 0.000000000000   ,  \"Imoff\" -> 0.000000000000   ,  \"στ1\" -> 0.000000000000   ,  \"στS\" -> 0.000000000000   ,  \"στN\" -> 0.000000000000    |>   , \r\"IDS0170_210310_RAW_cal__sam_\" ->   <|    \"ζ\" -> 0.012831327568   ,  \"τ1\" -> 0.013315909415   ,  \"τS\" -> 0.012590836847   ,  \"τN\" -> 0.000065003013   ,  \"τC\" -> 0.005276356243   ,  \"κ0\" -> 0.000000013610   ,  \"mm1\" -> 0.000047406274   ,  \"mm2\" -> 0.013137605540   ,  \"mm3\" -> 0.018225484932   ,  \"T\" -> 1.970000000000   ,  \"B\" -> 12.000000000000   ,  \"θ\" -> 0.000000000000   ,  \"Reoff\" -> 0.000000000000   ,  \"Imoff\" -> 0.000000000000   ,  \"στ1\" -> 0.000000000000   ,  \"στS\" -> 0.000000000000   ,  \"στN\" -> 0.000000000000    |>   , \r\"IDS0171_210310_RAW_cal__ref_\" ->   <|    \"ζ\" -> 0.024633693577   ,  \"τ1\" -> 0.014940694735   ,  \"τS\" -> 0.006137734482   ,  \"τN\" -> 0.000014567254   ,  \"τC\" -> 0.005080683927   ,  \"κ0\" -> 0.000000022488   ,  \"mm1\" -> 0.000067969819   ,  \"mm2\" -> 0.011256263587   ,  \"mm3\" -> 0.015001000908   ,  \"T\" -> 3.190000000000   ,  \"B\" -> 12.000000000000   ,  \"θ\" -> 0.000000000000   ,  \"Reoff\" -> 0.000000000000   ,  \"Imoff\" -> 0.000000000000   ,  \"στ1\" -> 0.000000000000   ,  \"στS\" -> 0.000000000000   ,  \"στN\" -> 0.000000000000    |>   , \r\"IDS0171_210310_RAW_cal__sam_\" ->   <|    \"ζ\" -> 0.019774146838   ,  \"τ1\" -> 0.013257273421   ,  \"τS\" -> 0.007064131508   ,  \"τN\" -> 0.000028000819   ,  \"τC\" -> 0.006942241845   ,  \"κ0\" -> 0.000000023477   ,  \"mm1\" -> 0.000068886863   ,  \"mm2\" -> 0.012935419574   ,  \"mm3\" -> 0.014427582022   ,  \"T\" -> 3.190000000000   ,  \"B\" -> 12.000000000000   ,  \"θ\" -> 0.000000000000   ,  \"Reoff\" -> 0.000000000000   ,  \"Imoff\" -> 0.000000000000   ,  \"στ1\" -> 0.000000000000   ,  \"στS\" -> 0.000000000000   ,  \"στN\" -> 0.000000000000    |>   , \r\"IDS0172_210310_RAW_cal__ref_\" ->   <|    \"ζ\" -> 0.027835388666   ,  \"τ1\" -> 0.013976390421   ,  \"τS\" -> 0.003539188638   ,  \"τN\" -> 0.000003774856   ,  \"τC\" -> 0.004420299329   ,  \"κ0\" -> 0.000000055482   ,  \"mm1\" -> 0.000054408485   ,  \"mm2\" -> 0.007998445403   ,  \"mm3\" -> 0.013985419121   ,  \"T\" -> 5.800000000000   ,  \"B\" -> 12.000000000000   ,  \"θ\" -> 0.000000000000   ,  \"Reoff\" -> 0.000000000000   ,  \"Imoff\" -> 0.000000000000   ,  \"στ1\" -> 0.000000000000   ,  \"στS\" -> 0.000000000000   ,  \"στN\" -> 0.000000000000    |>   , \r\"IDS0172_210310_RAW_cal__sam_\" ->   <|    \"ζ\" -> 0.029251354442   ,  \"τ1\" -> 0.014634751206   ,  \"τS\" -> 0.003873958746   ,  \"τN\" -> 0.000007000487   ,  \"τC\" -> 0.006827504775   ,  \"κ0\" -> 0.000000056438   ,  \"mm1\" -> 0.000072018576   ,  \"mm2\" -> 0.010723236476   ,  \"mm3\" -> 0.014661483476   ,  \"T\" -> 5.800000000000   ,  \"B\" -> 12.000000000000   ,  \"θ\" -> 0.000000000000   ,  \"Reoff\" -> 0.000000000000   ,  \"Imoff\" -> 0.000000000000   ,  \"στ1\" -> 0.000000000000   ,  \"στS\" -> 0.000000000000   ,  \"στN\" -> 0.000000000000    |>   , \r\"IDS0181_210310_RAW_cal__ref_\" ->   <|    \"ζ\" -> 0.196256884521   ,  \"τ1\" -> 0.071380539398   ,  \"τS\" -> 0.034448108903   ,  \"τN\" -> 0.119444210569   ,  \"τC\" -> 0.001245873609   ,  \"κ0\" -> 0.000000000908   ,  \"mm1\" -> 0.000199286041   ,  \"mm2\" -> 0.012356130491   ,  \"mm3\" -> 0.244165743118   ,  \"T\" -> 0.179000000000   ,  \"B\" -> 12.000000000000   ,  \"θ\" -> 90.000000000000   ,  \"Reoff\" -> -32111445.783132523300   ,  \"Imoff\" -> 0.000000000000   ,  \"στ1\" -> 0.005873597921   ,  \"στS\" -> 0.002285203630   ,  \"στN\" -> 0.000000000000    |>   , \r\"IDS0181_210310_RAW_cal__sam_\" ->   <|    \"ζ\" -> 0.161975781729   ,  \"τ1\" -> 0.073089805113   ,  \"τS\" -> 0.045018408115   ,  \"τN\" -> 0.161987434028   ,  \"τC\" -> 0.001482104484   ,  \"κ0\" -> 0.000000001038   ,  \"mm1\" -> 0.000201615809   ,  \"mm2\" -> 0.012976126678   ,  \"mm3\" -> 0.301929942357   ,  \"T\" -> 0.179000000000   ,  \"B\" -> 12.000000000000   ,  \"θ\" -> 90.000000000000   ,  \"Reoff\" -> 0.000000000000   ,  \"Imoff\" -> 0.000000000000   ,  \"στ1\" -> 0.000000000000   ,  \"στS\" -> 0.000000000000   ,  \"στN\" -> 0.000000000000    |>   , \r\"IDS0183_210310_RAW_cal__ref_\" ->   <|    \"ζ\" -> 0.374777480634   ,  \"τ1\" -> 0.116873786162   ,  \"τS\" -> 0.055337513541   ,  \"τN\" -> 0.665911779860   ,  \"τC\" -> 0.001012065497   ,  \"κ0\" -> 0.000000000453   ,  \"mm1\" -> 0.000273168605   ,  \"mm2\" -> 0.008156341144   ,  \"mm3\" -> 1.101013628401   ,  \"T\" -> 0.120000000000   ,  \"B\" -> 12.000000000000   ,  \"θ\" -> 90.000000000000   ,  \"Reoff\" -> -135984939.759036154000   ,  \"Imoff\" -> 0.000000000000   ,  \"στ1\" -> 0.014306498614   ,  \"στS\" -> 0.016176400349   ,  \"στN\" -> 0.000000000000    |>   , \r\"IDS0183_210310_RAW_cal__sam_\" ->   <|    \"ζ\" -> 0.300863384227   ,  \"τ1\" -> 0.104924004009   ,  \"τS\" -> 0.071070599729   ,  \"τN\" -> 0.992887187112   ,  \"τC\" -> 0.001721587800   ,  \"κ0\" -> 0.000000000548   ,  \"mm1\" -> 0.000392216822   ,  \"mm2\" -> 0.006637384427   ,  \"mm3\" -> 1.483679717825   ,  \"T\" -> 0.120000000000   ,  \"B\" -> 12.000000000000   ,  \"θ\" -> 90.000000000000   ,  \"Reoff\" -> 0.000000000000   ,  \"Imoff\" -> 0.000000000000   ,  \"στ1\" -> 0.000000000000   ,  \"στS\" -> 0.000000000000   ,  \"στN\" -> 0.000000000000    |>   , \r\"IDS0184_210310_RAW_cal__ref_\" ->   <|    \"ζ\" -> 0.262136034943   ,  \"τ1\" -> 0.088367137171   ,  \"τS\" -> 0.043836416470   ,  \"τN\" -> 0.254908544273   ,  \"τC\" -> 0.001163145607   ,  \"κ0\" -> 0.000000000664   ,  \"mm1\" -> 0.000237539268   ,  \"mm2\" -> 0.010917614909   ,  \"mm3\" -> 0.455431908812   ,  \"T\" -> 0.148000000000   ,  \"B\" -> 12.000000000000   ,  \"θ\" -> 90.000000000000   ,  \"Reoff\" -> -57475903.614457845700   ,  \"Imoff\" -> 0.000000000000   ,  \"στ1\" -> 0.008732968552   ,  
